vi "Main_Organizer.vi"() -> ()   [LabVIEW 2026]
doc: "Use this template to build a simple state machine design pattern. Each state executes code and determines which state to transition to."
uses:
  controls/UI Data.ctl
  controls/State.ctl
  <vilib>/Utility/miscctls.llb/LVPointTypeDef.ctl
panel:
  in  "Destination Folder":path
  in  "Original Files Folder":path
  in  "Bool_Erase":bool caption="Erase Originals"
  in  "Data":T1
  in  "Bol_State2":bool
  in  "Bol_Organize":bool
  in  "Exit":bool
  # "File Organizer Project\n1) Choose Original Files Folder\n2) Choose Destination Folder\n3) Set if need to erase originals"
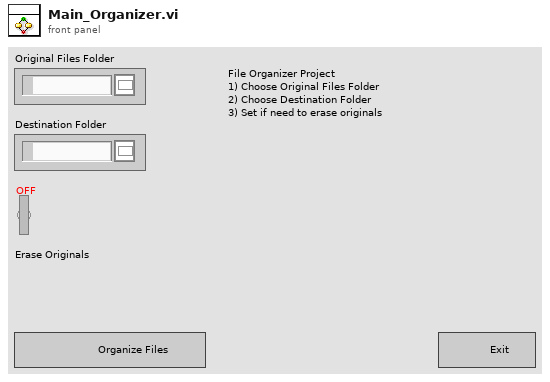
[diagram p1: front panel]
types:
  T1 = typedef "UI Data.ctl" = cluster{"Boolean":bool, "String":string, "Numeric":dbl}
  T2 = typedef "State.ctl" = enum16{"Initialize", "Wait for Event", "User State 1", "User State 2", "Exit"}
  T3 = typedef "LVPointTypeDef.ctl" = cluster{"Horizontal":i16, "Vertical":i16}
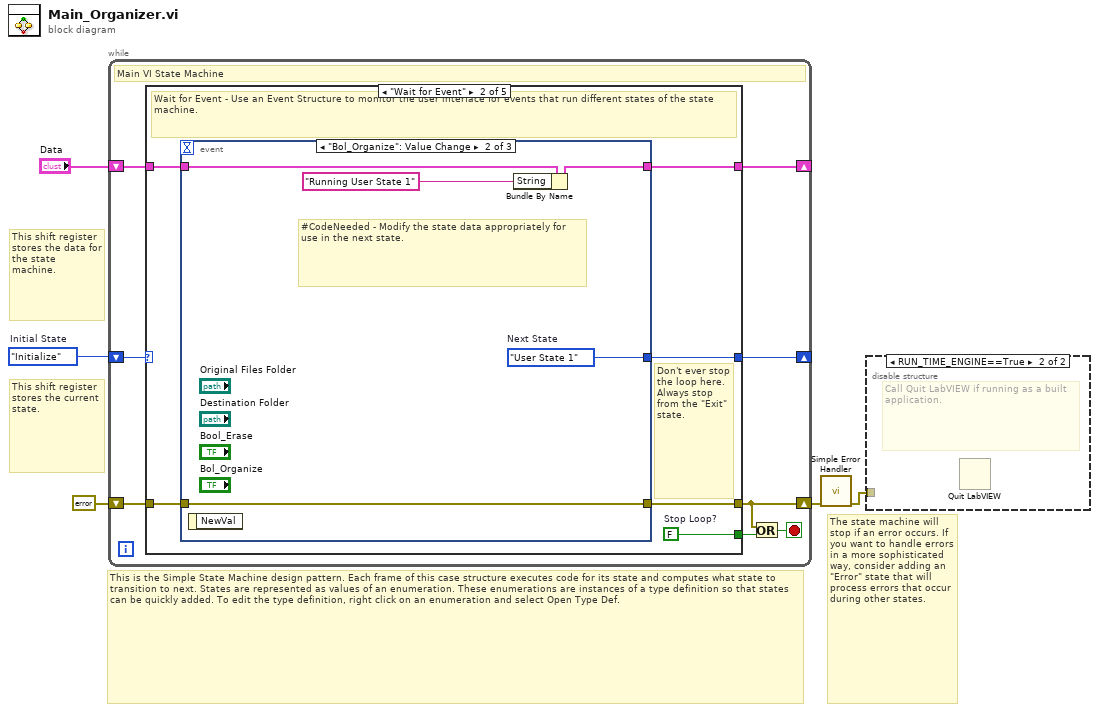
[diagram p0: block diagram]
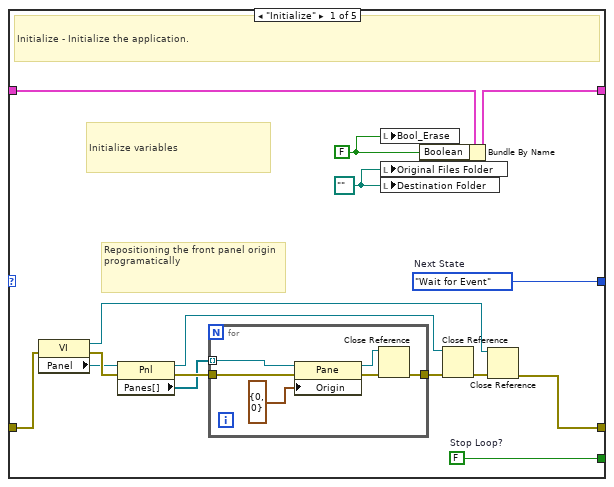
[diagram p3: hidden frame]
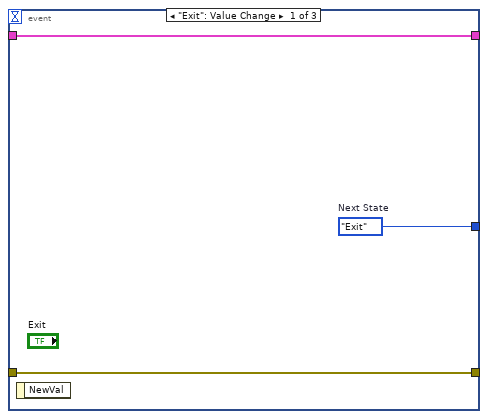
[diagram p4: hidden frame]
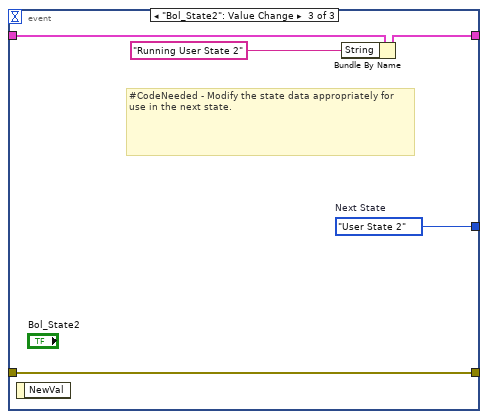
[diagram p5: hidden frame]
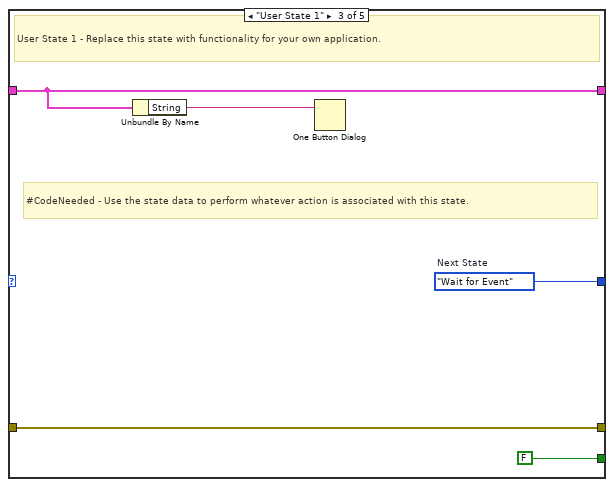
[diagram p6: hidden frame]
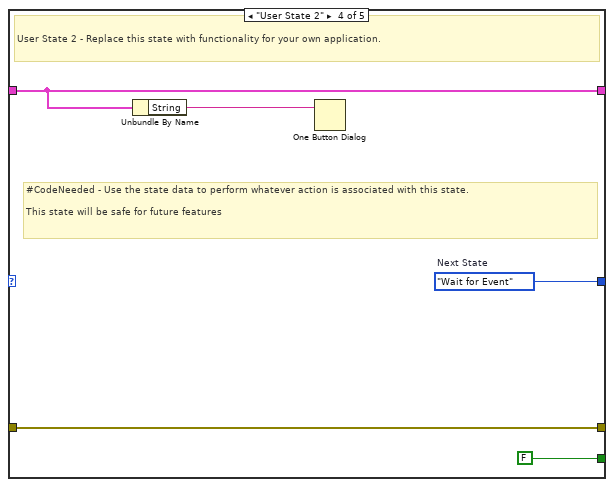
[diagram p7: hidden frame]
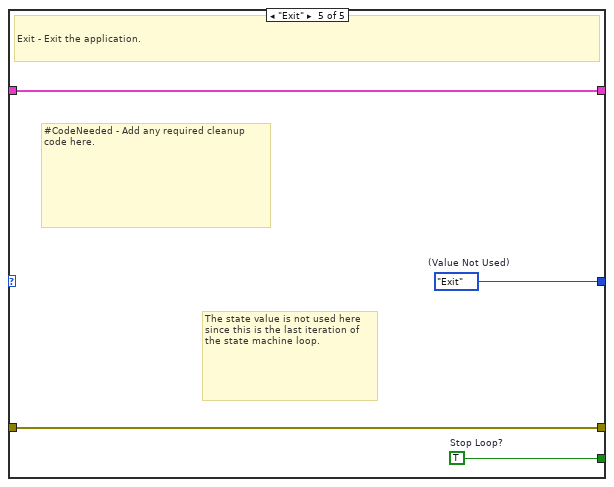
[diagram p8: hidden frame]
diagram:
  w5 = State."Initialize"  # Initial State
  # "The state machine will stop if an error occurs. If you want to handle errors in a more sophisticated way, consider adding an \"Error\" state that will process errors that occur during other states."
  # "This shift register stores the data for the state machine."
  # "This is the Simple State Machine design pattern. Each frame of this case structure executes code for its state and computes what state to transition to next. States are represented as values of an enumeration. These enumerations are instances of a type definition so that states can be quickly added. To edit the type definition, right click on an enumeration and select Open Type Def."
  # "This shift register stores the current state."
  n1 = while {
    shift-right: [w12] -> _
    shift-left: w5 -> [w13]
    shift-right: [w10] -> _
    shift-left: "Data" -> [w11]
    shift-right: [w6] -> w3
    shift-left: errorcluster {"status"=FALSE, "code"=0, "source"=""} ("error constant") -> [w9]
    stop <- w7 stop-if-true
    # "Main VI State Machine"
    n2 = case shown="\"Wait for Event\"" w13 {
      tunnel: [w29 w41 w59 w64 w68] -> w12
      tunnel: [w28 w40 FALSE ("Stop Loop?") FALSE ("Stop Loop?") w66] -> w8
      tunnel: w11 -> [w27 w39 w57 w62 w67]
      tunnel: [w26 w38 w57 w62 w67] -> w10
      tunnel: w9 -> [w24 w37 w55 w60 w65]
      tunnel: [w16 w36 w55 w60 w65] -> w6
      frame "Initialize" {
        w14 = path "" ("Original Files Folder")
        w25 = FALSE ("Replace_Me_Boolean")
        w28 = FALSE  # Stop Loop?
        w29 = State."Wait for Event"  # Next State
        # "Repositioning the front panel origin programatically"
        # "Initialize variables"
        # "Initialize - Initialize the application."
        n3 = property class="VI"(error in=w24) -> (reference out=w18:refnum<vi>, error out=w23:errorcluster, "Panel"=w22:refnum<vi>)  [unwired: 1 in]
        n4 = property class="Pnl"(reference=w22, error in=w23) -> (reference out=w17:refnum<vi>, error out=w21:errorcluster, "Panes[]"=w20:refnum<vi>[])
        n5 = for {
          tunnel: w21 -> [w34]
          tunnel: w20 -> [w35] mode=indexing
          tunnel: [w32] -> w15
          n6 = property class="Pane"(reference=w35, error in=w34, "Origin"=T3 {"Horizontal"=0, "Vertical"=0}) -> (reference out=w30:refnum<vi>, error out=w31:errorcluster)
          n7 = Close Reference(reference=w30, error in (no error)=w31) -> (error out=w32:errorcluster)
        }
        n8 = local write "Bool_Erase"(w25) -> ()
        n9 = local write "Original Files Folder"(w14) -> ()
        n10 = local write "Destination Folder"(w14) -> ()
        n11 = Bundle By Name(cluster=w27, "Boolean"=w25) -> (w26:T1)
        n12 = Close Reference(reference=w17, error in (no error)=w15) -> (error out=w19:errorcluster)
        n13 = Close Reference(reference=w18, error in (no error)=w19) -> (error out=w16:errorcluster)
      }
      frame "Wait for Event" {
        w40 = FALSE  # Stop Loop?
        # "Don't ever stop the loop here. Always stop from the \"Exit\" state."
        # "Wait for Event - Use an Event Structure to monitor the user interface for events that run different states of the state machine."
        n14 = event shown="[1] \"Bol_Organize\": Value Change" {
          selector: _ -> [_ _ _]
          dyn-events: _ -> [_ _ _]
          timeout: _ -> [_ _ _]
          tunnel: [w44 w49 w54] -> w41
          tunnel: w39 -> [w43 w48 w53]
          tunnel: [w43 w47 w52] -> w38
          tunnel: w37 -> [w42 w45 w50]
          tunnel: [w42 w45 w50] -> w36
          event "Exit": Value Change {
            w44 = State."Exit"  # Next State
            n15 = event-data() -> ()  [unwired: 1 in, 1 out]
          }
          event "Bol_Organize": Value Change {
            w49 = State."User State 1"  # Next State
            # "#CodeNeeded - Modify the state data appropriately for use in the next state."
            n16 = event-data() -> ()  [unwired: 1 in, 1 out]
            n17 = Bundle By Name(cluster=w48, "String"="Running User State 1" ("Running User State 1")) -> (w47:T1)
          }
          event "Bol_State2": Value Change {
            w54 = State."User State 2"  # Next State
            # "#CodeNeeded - Modify the state data appropriately for use in the next state."
            n18 = event-data() -> ()  [unwired: 1 in, 1 out]
            n19 = Bundle By Name(cluster=w53, "String"="Running User State 2" ("Running User State 2")) -> (w52:T1)
          }
        }
      }
      frame "User State 1" {
        w59 = State."Wait for Event"  # Next State
        # "#CodeNeeded - Use the state data to perform whatever action is associated with this state."
        # "User State 1 - Replace this state with functionality for your own application."
        n20 = Unbundle By Name(w57) -> ("String"=w56:string)
        n21 = One Button Dialog(message=w56) -> ()  [unwired: 1 in, 1 out]
      }
      frame "User State 2" {
        w64 = State."Wait for Event"  # Next State
        # "#CodeNeeded - Use the state data to perform whatever action is associated with this state.\n\nThis state will be safe for future features"
        # "User State 2 - Replace this state with functionality for your own application."
        n22 = Unbundle By Name(w62) -> ("String"=w61:string)
        n23 = One Button Dialog(message=w61) -> ()  [unwired: 1 in, 1 out]
      }
      frame "Exit" {
        w66 = TRUE  # Stop Loop?
        w68 = State."Exit"  # (Value Not Used)
        # "#CodeNeeded - Add any required cleanup code here."
        # "The state value is not used here since this is the last iteration of the state machine loop."
        # "Exit - Exit the application."
      }
    }
    n24 = Or(x=w6, y=w8) -> (x .or. y?=w7:bool)
  }
  n25 = call <vilib>:"Simple Error Handler.vi"("error in (no error)"=w3) -> ("error out"=w2:errorcluster)  [unwired: 4 in, 4 out]
  n26 = disable-structure shown="RUN_TIME_ENGINE==True" {
    disable-tunnel: w2 -> [_ _]
    frame condition #0 (active) {
    }
    frame condition #1 {
      # "Call Quit LabVIEW if running as a built application."
      n27 = Quit LabVIEW() -> ()  [unwired: 1 in]
    }
  }
